vi "create test channels.vi"() -> (0 "error out":errorcluster, 1 "names":string[](array[string]), 2 "Array":refnum<class "EthernetIP Channel.lvclass">[](array[class]), 3 "EthernetIP configuration out":refnum<class "EthernetIP configuration.lvclass">, 4 "2d":refnum<class "EthernetIP Channel.lvclass">[][](array[class]))   [LabVIEW 2013, in "EthernetIP tests.lvlib"]
uses:
  EthernetIP tests.lvlib
  channel/EthernetIP Channel.lvclass
  configuration/EthernetIP configuration.lvclass
  configuration/assembly definition.ctl
  configuration/assembly type.ctl
  <vilib>/NI/Tag Bus Module Framework/root configuration/TBM configuration.lvclass
panel:
  out "instances":T1[](array[typedef])
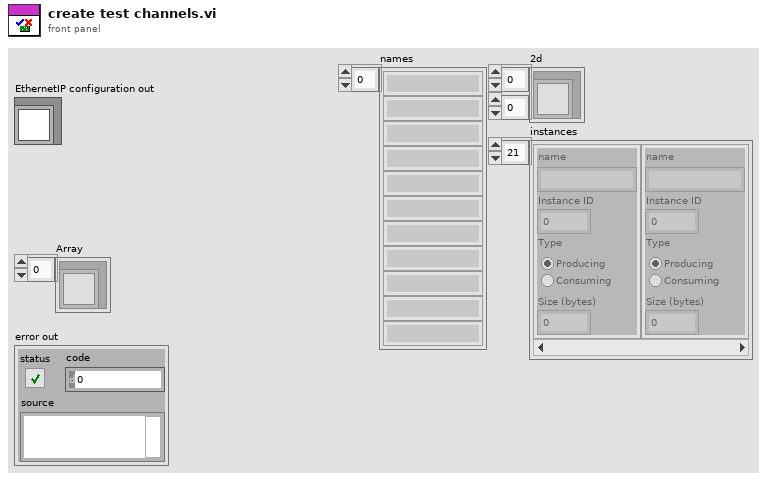
[diagram p1: front panel]
types:
  T1 = typedef "EthernetIP configuration.lvclass/assembly definition.ctl" = cluster{"name":string, "Instance ID":u32, "Type":T2, "Size (bytes)":u32}
  T2 = typedef "EthernetIP configuration.lvclass/assembly type.ctl" = enum32{"Producing", "Consuming"}
  T3 = typedef "tag bus.lvlib/tag descriptor.lvclass/Data Type.ctl" = enum16{"Double", "Single", "I64", "I32", "I16", "I8", "U64", "U32", "U16", "U8", "Boolean", "String", "Array of Double", "Array of Single", "Array of I64", "Array of I32", "Array of I16", "Array of I8", "Array of U64", "Array of U32", "Array of U16", "Array of U8", "Array of Boolean", "Array of String"}
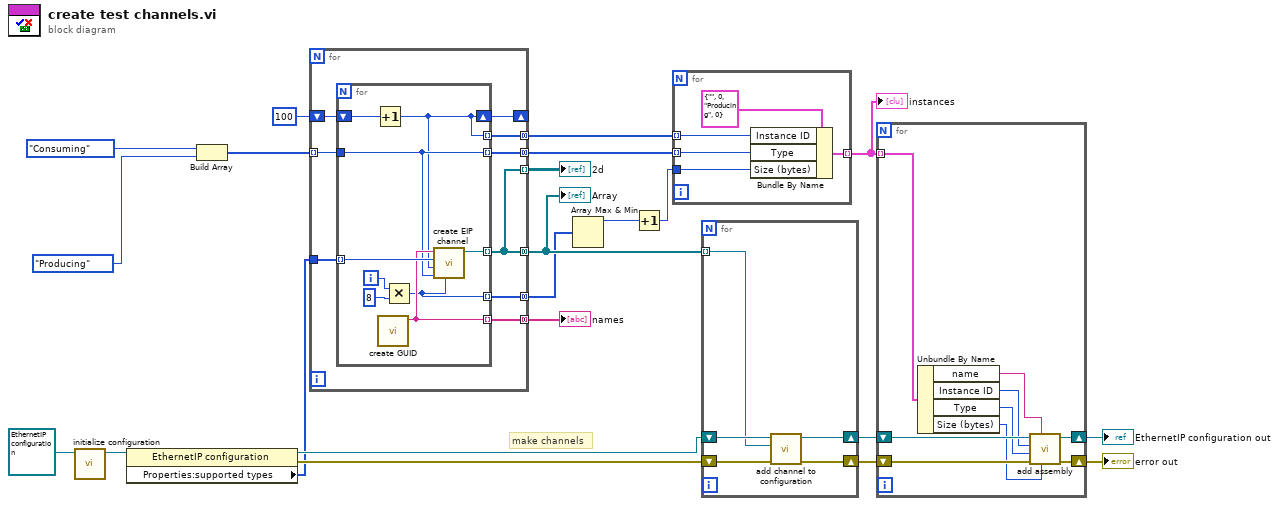
[diagram p0: block diagram]
diagram:
  # "make channels"
  n1 = call-dynamic "initialize configuration.vi"("configuration in"=refnum<class "EthernetIP configuration.lvclass"> refnum ("tag bus configurable plugin module configuration")) -> ("configuration out"=w20:refnum<class "EthernetIP configuration.lvclass">)  [unwired: 8 in, 2 out]
  n2 = property class="EthernetIP configuration"(reference=w20) -> (reference out=w16:refnum<class "EthernetIP configuration.lvclass">, error out=w19:errorcluster, "Properties:supported types"=w15:T3[])  [unwired: 1 in]
  n3 = Build Array(assembly_type."Consuming" ("Type"), assembly_type."Producing" ("Type")) -> (w14:T2[])
  n4 = for {
    tunnel: w14 -> [w31] mode=indexing
    tunnel: [w28] -> w18 mode=concatenating
    tunnel: w15 -> [w30]
    tunnel: [w29] -> w13 mode=concatenating
    tunnel: [w28] -> w12 mode=indexing
    tunnel: [w27] -> w10 mode=concatenating
    tunnel: [w26] -> w11 mode=concatenating
    tunnel: [w25] -> w8 mode=concatenating
    shift-right: [w23] -> _
    shift-left: 100 -> [w24]
    n5 = for {
      tunnel: w31 -> [w34]
      tunnel: [w40] -> w28 mode=indexing
      tunnel: w30 -> [w39] mode=indexing
      tunnel: [w37] -> w29 mode=indexing
      tunnel: [w32] -> w27 mode=indexing
      tunnel: [w36] -> w26 mode=indexing
      tunnel: [w34] -> w25 mode=indexing
      shift-right: [w32] -> w23
      shift-left: w24 -> [w33]
      i -> [w35]
      n6 = Increment(x=w33) -> (x+1=w32:i32)
      n7 = call <vilib>:"create GUID.vi"() -> ("uuid"=w37:string)  [unwired: 11 in]
      n8 = Multiply(x=w35, y=8) -> (x*y=w36:i32)
      n9 = call "create EIP channel.vi"("byte index"=w36, "Type"=w34, "Instance ID"=w32, "data type"=w39, "name"=w37) -> ("EthernetIP Channel out"=w40:refnum<class "EthernetIP Channel.lvclass">)  [unwired: 6 in]
    }
  }
  "Array" <- w18
  "names" <- w13
  "2d" <- w12
  n10 = Array Max & Min(array=w11) -> (max value=w9:i32)  [unwired: 3 out]
  n11 = Increment(x=w9) -> (x+1=w7:i32)
  n12 = for {
    tunnel: w10 -> [w42] mode=indexing
    tunnel: w7 -> [w44]
    tunnel: w8 -> [w43] mode=indexing
    tunnel: [w41] -> w5 mode=indexing
    n13 = Bundle By Name(cluster=T1 {"name"="", "Instance ID"=0, "Type"=enum."Producing", "Size (bytes)"=0} ("assembly definition"), "Instance ID"=w42, "Type"=w43, "Size (bytes)"=w44) -> (w41:T1)
  }
  "instances" <- w5
  n14 = for {
    tunnel: w18 -> [w48] mode=indexing
    shift-right: [w47] -> w4
    shift-left: w16 -> [w50]
    shift-right: [w46] -> w3
    shift-left: w19 -> [w49]
    n15 = call "add channel to configuration.vi"("error in"=w49, "TBM channel in"=w48, "EthernetIP configuration in"=w50) -> ("error out"=w46:errorcluster, "EthernetIP configuration out"=w47:refnum<class "EthernetIP configuration.lvclass">)  [unwired: 7 in]
  }
  n16 = for {
    tunnel: w5 -> [w55] mode=indexing
    shift-right: [w56] -> w1
    shift-left: w4 -> [w59]
    shift-right: [w57] -> w2
    shift-left: w3 -> [w58]
    n17 = Unbundle By Name(w55) -> ("name"=w54:string, "Instance ID"=w53:u32, "Type"=w52:T2, "Size (bytes)"=w51:u32)
    n18 = call "add assembly.vi"("size (bytes)"=w51, "name"=w54, "error in"=w58, "Type"=w52, "instance ID"=w53, "EthernetIP configuration in"=w59) -> ("error out"=w57:errorcluster, "EthernetIP configuration out"=w56:refnum<class "EthernetIP configuration.lvclass">)  [unwired: 4 in]
  }
  "error out" <- w2
  "EthernetIP configuration out" <- w1
